vi "I2C Device Read.vi"(0 "handle":u32, 5 "Slave device address":u32, 7 "Size to transfer":u32, 9 "options":T1, 11 "error in (no error)":errorcluster) -> (4 "handle out":u32, 6 "Data read":u8[](array[numeric]) format="%.0x", 8 "buffer":string, 10 "sizeTransfered":u32, 15 "error out":errorcluster)   [LabVIEW 2017, in "libMPSSE.lvlib"]
doc: "FTDI_API FT_STATUS I2C_DeviceRead(FT_HANDLE handle, uint32 deviceAddress, \nuint32 sizeToTransfer, uint8 *buffer, uint32 *sizeTransfered, uint32 options);\n\nOptions\nThis parameter specifies data transfer options. The bit positions defined for each of these options are:\n\nBIT0: if set then a start condition is generated in the I2C bus before the transfer begins. A bit mask is defined for this options in file ftdi_i2c.h as I2C_TRANSFER_OPTIONS_START_BIT\n\nBIT1: if set then a stop condition is generated in the I2C bus after the transfer ends. A bit mask is defined for this options in file ftdi_i2c.h as I2C_TRANSFER_OPTIONS_STOP_BIT\n\nBIT2: if set then the function will return when a device nAcks after a byte has been transferred. If not set then the function will continue transferring the stream of bytes even if the device nAcks. A bit mask is defined for this options in file ftdi_i2c.h as I2C_TRANSFER_OPTIONS_BREAK_ON_NACK\n\nBIT3: reserved (only used in I2C_DeviceRead)\n\nBIT4: setting this bit will invoke a multi byte I2C\nApplication Note: AN_177 User Guide For libMPSSE – I2C Version 1.4 Document Reference No.: FT_000466 Clearance No.: FTDI# 210 11 Copyright © 2011 Future Technology Devices International Limited\ntransfer without having delays between the START, ADDRESS, DATA and STOP phases. Size of the transfer in parameters sizeToTransfer and sizeTransfered are in bytes. The bit mask defined for this bit is I2C_TRANSFER_OPTIONS_FAST_TRANSFER_BYTES*\n\nBIT5: setting this bit would invoke a multi bit transfer without having delays between the START, ADDRESS, DATA and STOP phases. Size of the transfer in parameters sizeToTransfer and sizeTransfered are in bytes. The bit mask defined for this bit is I2C_TRANSFER_OPTIONS_FAST_TRANSFER_BITS*\n\nBIT6: the deviceAddress parameter is ignored if this bit is set. This feature may be useful in generating a special I2C bus conditions that do not require any address to be passed.Setting this bit is effective only when either I2C_TRANSFER_OPTIONS_FAST_TRANSFER_BYTES or I2C_TRANSFER_OPTIONS_FAST_TRANSFER_BITS is set. The bit mask defined for this bit is I2C_TRANSFER_OPTIONS_NO_ADDRESS*\n\nBIT7 – BIT31: reserved"
uses:
  libMPSSE.lvlib
  libMPSSE-SPI-LabVIEW-master/libMPSSE.dll
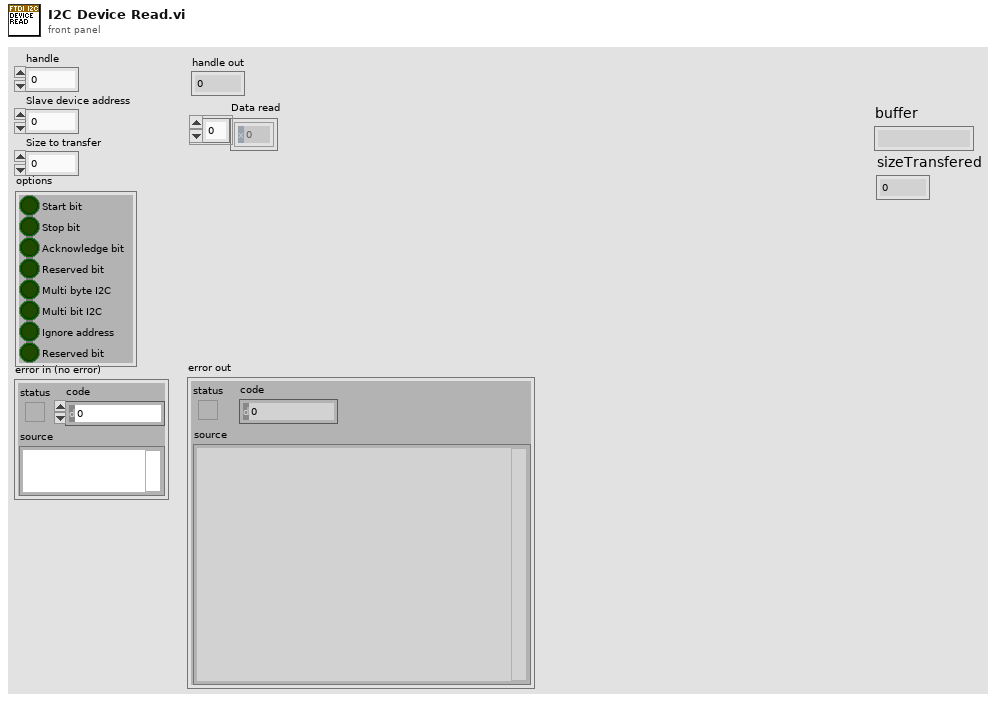
[diagram p1: front panel]
types:
  T1 = cluster{"Start bit":bool, "Stop bit":bool, "Acknowledge bit":bool, "Reserved bit":bool, "Multi byte I2C":bool, "Multi bit I2C":bool, "Ignore address":bool, "Reserved bit":bool}
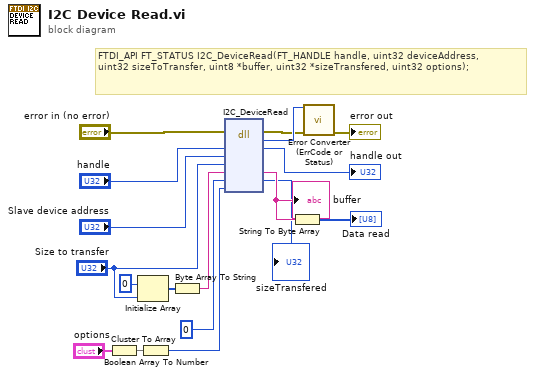
[diagram p0: block diagram]
diagram:
  # "FTDI_API FT_STATUS I2C_DeviceRead(FT_HANDLE handle, uint32 deviceAddress, \nuint32 sizeToTransfer, uint8 *buffer, uint32 *sizeTransfered, uint32 options);"
  n1 = Cluster To Array(cluster="options") -> (array=w7:bool[])
  n2 = Initialize Array(u8 0, "Size to transfer") -> (w10:u8[])
  n3 = Boolean Array To Number(Boolean array=w7) -> (number=w6:u32)
  n4 = Byte Array To String(unsigned byte array=w10) -> (string=w9:string)
  n5 = dll-call lib="\\\\Mac\\Home/Desktop/libMPSSE-SPI-LabVIEW-master/libMPSSE.dll" fn="I2C_DeviceRead"(error in="error in (no error)", "handle"="handle", "deviceAddress"="Slave device address", "sizeToTransfer"="Size to transfer", "buffer"=w9, "sizeTransfered"=u32 0, "options"=w6) -> (error out=w12:errorcluster, "return type"=w18:u32, "handle"=→"handle out":u32, "buffer"=w3:string, "sizeTransfered"=→"sizeTransfered":u32)  [unwired: 5 in, 1 out]
  "buffer" <- w3
  n6 = String To Byte Array(string=w3) -> (unsigned byte array=→"Data read":u8[])
  n7 = call "Error Converter (ErrCode or Status).vi"("error code"=w18, "error in (no error)"=w12) -> ("error out"=→"error out":errorcluster)  [unwired: 13 in]
